vi "ccidinfo-r.vi"(1 "Data Type":T1, 2 "Slot":T2) -> (0 "Data":string)   [LabVIEW 2013]
uses:
  SystemCode/SysControl/Slot.ctl
  CCID info.ctl
  GlobalValue.vi
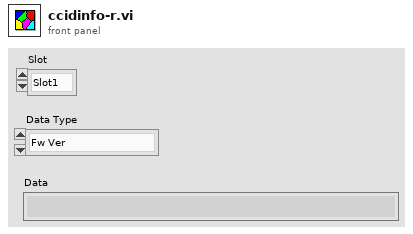
[diagram p1: front panel]
types:
  T1 = typedef "CCID info.ctl" = enum16{"Fw Ver", "HW Ver", "CCID", "WiFiName", "DevID"}
  T2 = typedef "Slot.ctl" = enum16{"Slot1", "Slot2", "Slot3", "Slot4"}
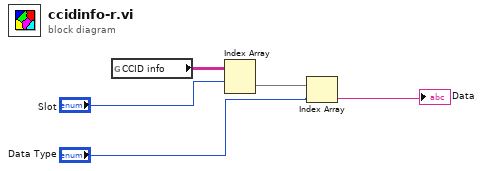
[diagram p0: block diagram]
diagram:
  n1 = global read "GlobalValue.vi" "CCID info"() -> (w5:string[][])
  n2 = Index Array(array=w5, index (row)="Slot") -> (element=w3:string[])  [unwired: 1 in]
  n3 = Index Array(array=w3, index="Data Type") -> (element=→"Data":string)
